vi "State Set.vi"(8 "error in (no error)":errorcluster caption="错误输入（无错误）", 11 "ScreenSwitching 输入":refnum<class "Screen Switching.lvclass">) -> (0 "error out":errorcluster caption="错误输出", 3 "ScreenSwitching 输出":refnum<class "Screen Switching.lvclass">)   [LabVIEW 2016, in "Screen Switching.lvlib" / "Screen Switching.lvclass"]
uses:
  Screen Switching.lvclass
  Screen Switching.lvclass/Screen Switching.ctl
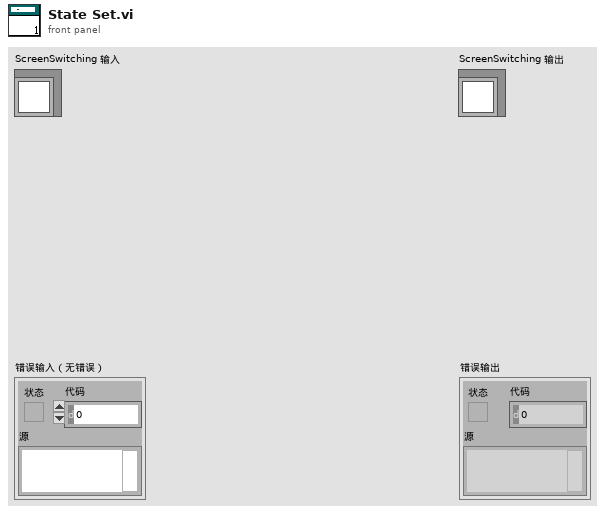
[diagram p1: front panel]
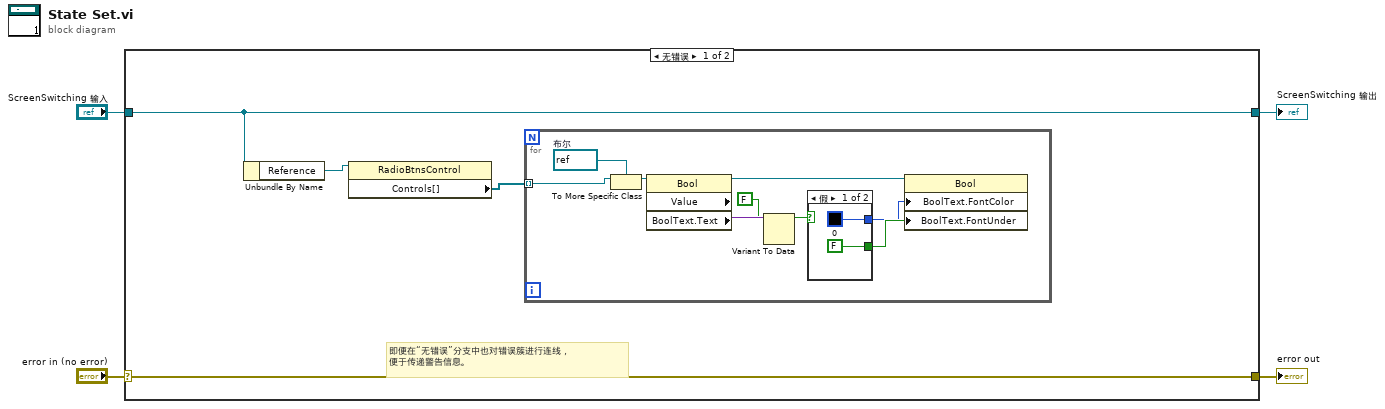
[diagram p0: block diagram]
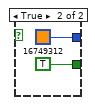
[diagram p2: hidden frame]
diagram:
  n1 = case shown="无错误" "error in (no error)" {
    selector: "error in (no error)" -> [w8 w23]
    tunnel: [w8 w23] -> w3
    tunnel: [w6 w22] -> w1
    tunnel: "ScreenSwitching 输入" -> [w6 w22]
    frame No Error {
      # "即便在“无错误”分支中也对错误簇进行连线，\n便于传递警告信息。"
      n2 = Unbundle By Name(w6) -> ("Reference"=w5:refnum<vi>)
      n3 = property class="RadioBtnsControl"(reference=w5) -> ("Controls[]"=w7:refnum<vi>[])  [unwired: 1 in, 2 out]
      n4 = for {
        tunnel: w7 -> [w17] mode=indexing
        w16 = refnum<vi> refnum  # 布尔
        n5 = To More Specific Class(target class=w16, reference=w17) -> (specific class reference=w15:refnum<vi>)  [unwired: 1 in, 1 out]
        n6 = property class="Bool" props=["Value", "BoolText", "Text"](reference=w15) -> (reference out=w11:refnum<vi>, "Value"=w14:variant)  [unwired: 1 in, 2 out]
        n7 = Variant To Data(type=FALSE, Variant=w14) -> (data=w12:bool)  [unwired: 1 in, 1 out]
        n8 = case shown="假" w12 {
          tunnel: [FALSE TRUE] -> w10
          tunnel: [u32 0 ("布尔文本.字体:颜色") u32 16749312 ("布尔文本.字体:颜色")] -> w9
          frame False {
          }
          frame True {
          }
        }
        n9 = property class="Bool"(reference=w11, "BoolText.FontColor"=w9, "BoolText.FontUnder"=w10) -> ()  [unwired: 1 in, 2 out]
      }
    }
    frame Error {
    }
  }
  "error out" <- w3
  "ScreenSwitching 输出" <- w1
